vi "Punto_3.vi"() -> ()   [LabVIEW 2019]
panel:
  in  "SELECTOR":bool
  out "Decremento":bool
  out "Incremento":bool
  in  "Temp Mín":dbl=25.0
  in  "Temp Máx":dbl=200.0
  in  "Decremento T":i32(knob) scale=0.0..10.0
  in  "Incremento T":i16(knob) scale=0.0..10.0
  in  "RATA DE T(°C/Seg)":i32(knob) scale=1.0..10.0
  out "Sensor de Temperatura °C":dbl(slide) scale=0.0..200.0
  # "DECREMENTAR"
  # "INCREMENTAR"
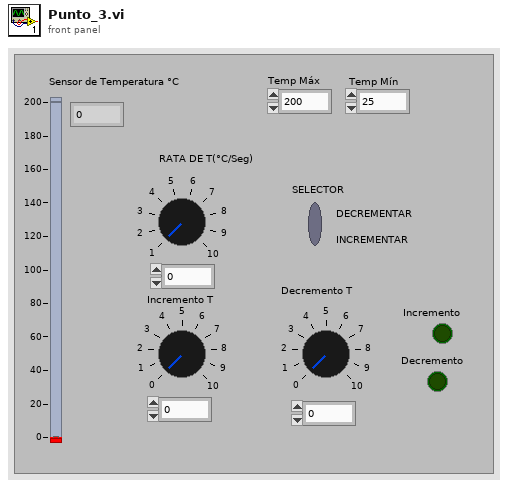
[diagram p1: front panel]
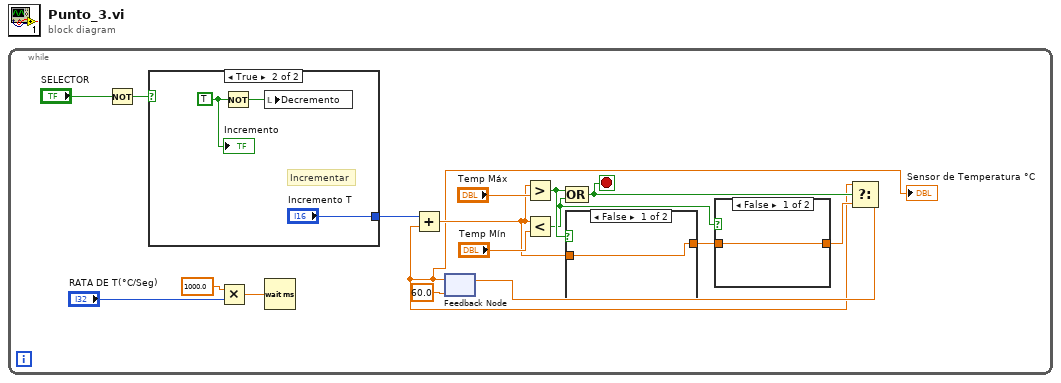
[diagram p0: block diagram]
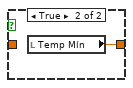
[diagram p2: hidden frame]
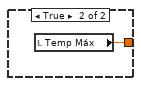
[diagram p3: hidden frame]
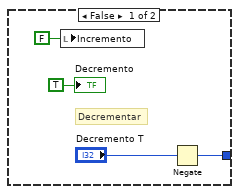
[diagram p4: hidden frame]
diagram:
  n1 = while {
    stop <- w2 stop-if-true
    n2 = Not(x="SELECTOR") -> (.not. x?=w10:bool)
    n3 = case shown="True" w10 {
      tunnel: [w24 "Incremento T"] -> w15
      frame False {
        # "Decrementar"
        n4 = local write "Incremento"(FALSE ("Decremento")) -> ()
        n5 = Negate(x="Decremento T") -> (-x=w24:i32)
        "Decremento" <- TRUE ("Decremento")
      }
      frame True {
        w27 = TRUE ("Incremento")
        # "Incrementar"
        n6 = Not(x=w27) -> (.not. x?=w26:bool)
        n7 = local write "Decremento"(w26) -> ()
        "Incremento" <- w27
      }
    }
    n8 = Multiply(x=1000.0 ("y"), y="RATA DE T(°C/Seg)") -> (x*y=w14:dbl)
    n9 = Wait (ms)(milliseconds to wait=w14) -> ()  [unwired: 1 out]
    n10 = feedback #1(60.0) -> (w1:dbl)
    "Sensor de Temperatura °C" <- w1
    n11 = Add(x=w15, y=w1) -> (x+y=w4:dbl)
    n12 = Greater?(x=w4, y="Temp Máx") -> (0:w8:bool)
    n13 = Less?(x=w4, y="Temp Mín") -> (x < y?=w7:bool)
    n14 = Compound Arithmetic op=OR(w8, w7) -> (w2:bool)
    n15 = case shown="False" w8 {
      tunnel: w4 -> [w20 _]
      tunnel: [w20 w21] -> w6
      frame False {
      }
      frame True {
        n16 = local read "Temp Máx"() -> (w21:dbl)
      }
    }
    n17 = case shown="False" w7 {
      tunnel: w6 -> [w18 _]
      tunnel: [w18 w19] -> w5
      frame False {
      }
      frame True {
        n18 = local read "Temp Mín"() -> (w19:dbl)
      }
    }
    n19 = Select(t=w1, s=w2, f=w5) -> (s? t:f=w3:dbl)
    n20 = feedback-in #1(w3) -> ()
  }
